vi "Set_Test_Data_Rows.vi"(9 "输入行数据":string[](array[string]), 10 "索引 (行)":i32, 11 "测试数据 2":refnum<vi>) -> (1 "数组":string[](array[string]), 3 "引用输出":refnum<vi>)   [LabVIEW 2018]
panel:
  out "error out":errorcluster caption="错误输出"
  in  "error in (no error)":errorcluster caption="错误输入（无错误）"
  out "数值":i32
  in  "测试数据":i32(listbox)
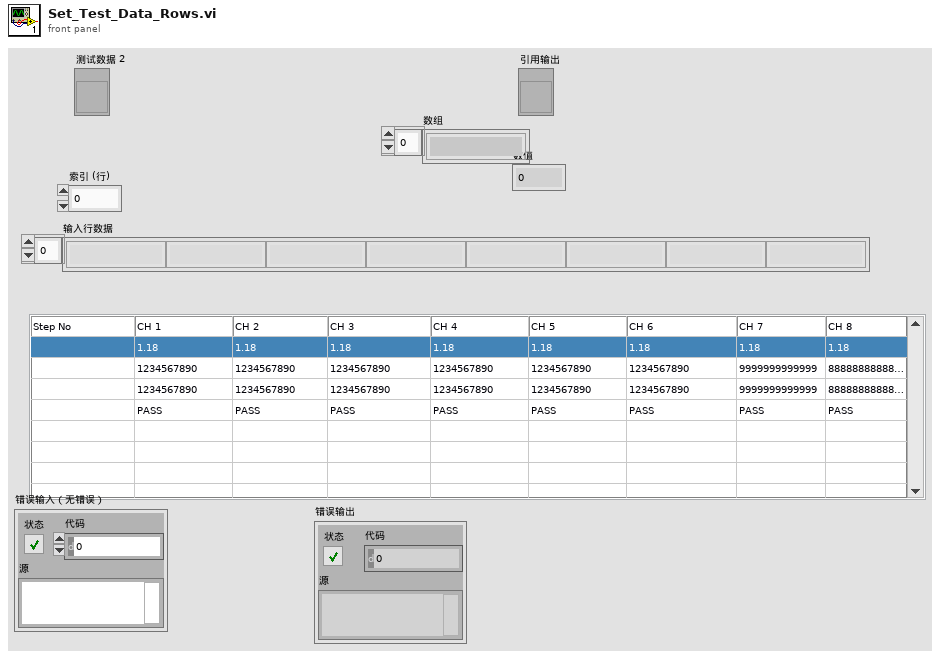
[diagram p1: front panel]
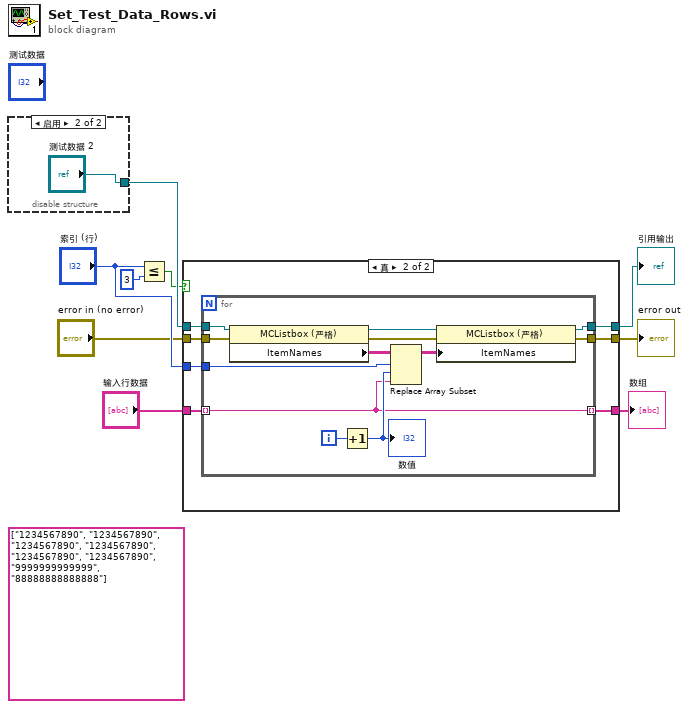
[diagram p0: block diagram]
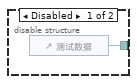
[diagram p2: hidden frame]
diagram:
  (unwired) string[] ["1234567890", "1234567890", "1234567890", "1234567890", "1234567890", "1234567890", "9999999999999", "88888888888888"]
  n1 = disable-structure shown="启用" {
    disable-tunnel: [w10 "测试数据 2"] -> w9
    frame Disabled {
      n2 = control-ref of="测试数据"() -> (w10:refnum<vi>)
    }
    frame Enabled {
    }
  }
  n3 = Less Or Equal?(x="索引 (行)", y=3) -> (x <= y?=w8:bool)
  n4 = case shown="真" w8 {
    tunnel: w9 -> [w13 w20]
    tunnel: "输入行数据" -> [_ w19]
    tunnel: "索引 (行)" -> [_ w18]
    tunnel: [w13 w17] -> w4
    tunnel: "error in (no error)" -> [w12 w16]
    tunnel: [w12 w15] -> w2
    tunnel: [_ w14] -> w1
    frame False {
    }
    frame True {
      n5 = for {
        tunnel: w20 -> [w31]
        tunnel: w19 -> [w21] mode=indexing
        tunnel: w18 -> [w30]
        tunnel: [w25] -> w17
        tunnel: w16 -> [w24]
        tunnel: [w23] -> w15
        tunnel: [w21] -> w14 mode=indexing
        i -> [w27]
        n6 = property class="MCListbox (严格)"(reference=w31, error in=w24) -> (reference out=w32:refnum<vi>, error out=w22:errorcluster, "ItemNames"=w29:string[][])
        n7 = Increment(x=w27) -> (x+1=w28:i32)
        "数值" <- w28
        n8 = Replace Array Subset(array=w29, new element=w21, index (row)=w30, index (col)=w28) -> (w26:string[][])
        n9 = property class="MCListbox (严格)"(reference=w32, error in=w22, "ItemNames"=w26) -> (reference out=w25:refnum<vi>, error out=w23:errorcluster)
      }
    }
  }
  "引用输出" <- w4
  "error out" <- w2
  "数组" <- w1
